vi "Configure Ramp.vi"(0 "VISA resource name":refnum<visa-resource-name>, 5 "Loop (0: 1)":u16(ring) items=["1", "2"], 7 "Rate Value (0.1)":dbl=0.1 min=0.0 max=100.0 step=0.1 format="%.1f", 9 "Ramping On/Off (F: Off)":bool, 11 "error in (no error)":errorcluster) -> (4 "VISA resource name out":refnum<visa-resource-name>, 15 "error out":errorcluster)   [LabVIEW 2019, in "Lake Shore Cryotronics 331.lvlib"]
doc: "This VI configures the parameters of a control loop's ramp."
uses:
  <instrlib>/Lake Shore Cryotronics 331/Lake Shore Cryotronics 331.lvlib
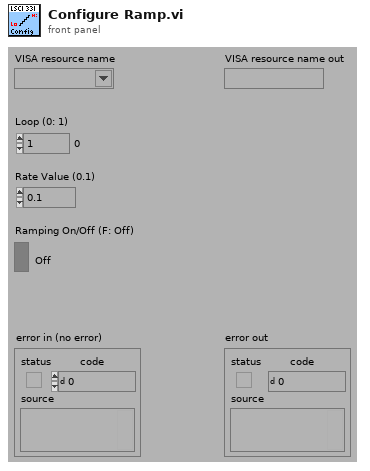
[diagram p1: front panel]
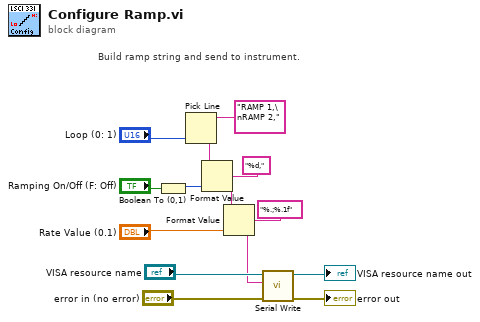
[diagram p0: block diagram]
diagram:
  # "Build ramp string and send to instrument."
  n1 = Boolean To (0,1)(Boolean="Ramping On/Off (F: Off)") -> (0, 1=w11:i16)
  n2 = Pick Line(multi-line string="RAMP 1,\nRAMP 2,", line index="Loop (0: 1)") -> (output string=w9:string)  [unwired: 1 in]
  n3 = Format Value(string ("")=w9, format string="%d,", value (0)=w11) -> (output string=w6:string)
  n4 = Format Value(string ("")=w6, format string="%.;%.1f", value (0)="Rate Value (0.1)") -> (output string=w1:string)
  n5 = call <instrlib>:"Serial Write.vi"("error in (no error)"="error in (no error)", "Write Buffer (\"\")"=w1, "VISA resource name"="VISA resource name") -> ("error out"=→"error out":errorcluster, "VISA resource name out"=→"VISA resource name out":refnum<visa-resource-name>)  [unwired: 6 in, 1 out]
